vi "WLAN Tx Test Get Default USL.vi"(8 "error in (no error)":errorcluster, 11 "Template Tx Test in":refnum<class "niDTS WLAN Tx Test.lvclass">) -> (0 "error out":errorcluster, 2 "Default USL":T1 {"OBW"."Stop Frequency (Hz)" format="%#_4p"; "OBW"."Start Frequency (Hz)" format="%#_4p"; "OBW"."OBW (Hz)" format="%#_4p"}, 3 "Template Tx Test out":refnum<class "niDTS WLAN Tx Test.lvclass">)   [LabVIEW 2015, in "niDTS WLAN.lvlib" / "niDTS WLAN Tx Test.lvclass"]
uses:
  niDTS WLAN Tx Test.lvclass
  Includes/niDTS WLAN Tx Test INC Results.ctl
  Includes/niDTS WLAN Tx Test INC MOD EVM Results.ctl
  Includes/Results/niDTS Tx RES INC EVM.ctl
  Includes/niDTS WLAN Tx Test INC TXP Results.ctl
  Includes/niDTS WLAN Tx Test INC TXP Result SINGLE.ctl
  Includes/niDTS WLAN Tx Test INC OBW Results.ctl
  Instrument/INSTR TX/Results/niDTS WLAN INSTR TX INC SEM Results.ctl
  Instrument/INSTR TX/Results/niDTS WLAN INSTR TX INC SEM FSEGemts Results.ctl
  Includes/Results/niDTS Tx RES INC SEM FSEGemts.ctl
  Instrument/INSTR TX/Results/niDTS WLAN INSTR TX INC SEM MARGin Results.ctl
  Includes/Results/niDTS Tx RES INC SEM Margin.ctl
  Instrument/INSTR TX/Results/niDTS WLAN INSTR TX INC OFDM Impairments Results.ctl
  niDTS WLAN Tx Test.lvclass/niDTS WLAN Tx Test.ctl
  Includes/niDTS WLAN Tx Test INC Default Limits.vi
  niDTS WLAN.lvlib
  Instrument/INSTR TX/niDTS WLAN INSTR TX.lvclass
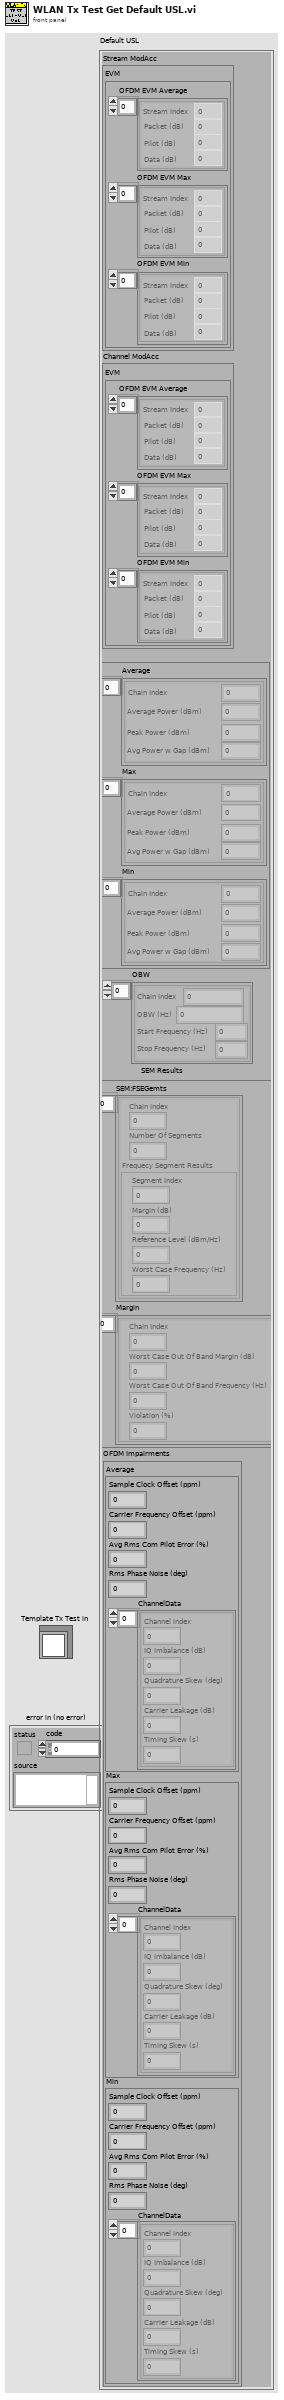
[diagram p1: front panel]
types:
  T1 = typedef "niDTS WLAN.lvlib/niDTS WLAN Tx Test INC Results.ctl" = cluster{"Stream ModAcc":T2, "Channel ModAcc":T2, "TXP":T4, "OBW":T6[], "SEM Results":T7, "OFDM Impairments":T12}
  T2 = typedef "niDTS WLAN.lvlib/niDTS WLAN Tx Test INC MOD EVM Results.ctl" = cluster{"EVM":cluster{"OFDM EVM Average":T3[], "OFDM EVM Max":T3[], "OFDM EVM Min":T3[]}}
  T3 = typedef "niDTS WLAN.lvlib/niDTS Tx RES INC EVM.ctl" = cluster{"Stream Index":i32, "Packet (dB)":dbl, "Pilot (dB)":dbl, "Data (dB)":dbl}
  T4 = typedef "niDTS WLAN.lvlib/niDTS WLAN Tx Test INC TXP Results.ctl" = cluster{"Average":T5[], "Max":T5[], "Min":T5[]}
  T5 = typedef "niDTS WLAN.lvlib/niDTS WLAN Tx Test INC TXP Result SINGLE.ctl" = cluster{"Chain Index":dbl, "Average Power (dBm)":dbl, "Peak Power (dBm)":dbl, "Avg Power w Gap (dBm)":dbl}
  T6 = typedef "niDTS WLAN.lvlib/niDTS WLAN Tx Test INC OBW Results.ctl" = cluster{"Chain Index":dbl, "OBW (Hz)":dbl, "Start Frequency (Hz)":dbl, "Stop Frequency (Hz)":dbl}
  T7 = typedef "niDTS WLAN.lvlib/niDTS WLAN INSTR TX.lvclass/niDTS WLAN INSTR TX INC SEM Results.ctl" = cluster{"SEM:FSEGemts":T8, "Margin":T10}
  T8 = typedef "niDTS WLAN.lvlib/niDTS WLAN INSTR TX.lvclass/niDTS WLAN INSTR TX INC SEM FSEGemts Results.ctl" = T9[]
  T9 = typedef "niDTS WLAN.lvlib/niDTS Tx RES INC SEM FSEGemts.ctl" = cluster{"Chain Index":i32, "Number Of Segments":i32, "Frequecy Segment Results":cluster{"Segment Index":i32, "Margin (dB)":dbl, "Reference Level (dBm/Hz)":dbl, "Worst Case Frequency (Hz)":dbl}}
  T10 = typedef "niDTS WLAN.lvlib/niDTS WLAN INSTR TX.lvclass/niDTS WLAN INSTR TX INC SEM MARGin Results.ctl" = T11[]
  T11 = typedef "niDTS WLAN.lvlib/niDTS Tx RES INC SEM Margin.ctl" = cluster{"Chain Index":i32, "Worst Case Out Of Band Margin (dB)":dbl, "Worst Case Out Of Band Frequency (Hz)":dbl, "Violation (%)":dbl}
  T12 = typedef "niDTS WLAN.lvlib/niDTS WLAN INSTR TX.lvclass/niDTS WLAN INSTR TX INC OFDM Impairments Results.ctl" = cluster{"Average":cluster{"Sample Clock Offset (ppm)":dbl, "Carrier Frequency Offset (ppm)":dbl, "Avg Rms Com Pilot Error (%)":dbl, "Rms Phase Noise (deg)":dbl, "ChannelData":cluster{"Channel Index":i32, "IQ Imbalance (dB)":dbl, "Quadrature Skew (deg)":dbl, "Carrier Leakage (dB)":dbl, "Timing Skew (s)":dbl}[]}, "Max":cluster{"Sample Clock Offset (ppm)":dbl, "Carrier Frequency Offset (ppm)":dbl, "Avg Rms Com Pilot Error (%)":dbl, "Rms Phase Noise (deg)":dbl, "ChannelData":cluster{"Channel Index":i32, "IQ Imbalance (dB)":dbl, "Quadrature Skew (deg)":dbl, "Carrier Leakage (dB)":dbl, "Timing Skew (s)":dbl}[]}, "Min":cluster{"Sample Clock Offset (ppm)":dbl, "Carrier Frequency Offset (ppm)":dbl, "Avg Rms Com Pilot Error (%)":dbl, "Rms Phase Noise (deg)":dbl, "ChannelData":cluster{"Channel Index":i32, "IQ Imbalance (dB)":dbl, "Quadrature Skew (deg)":dbl, "Carrier Leakage (dB)":dbl, "Timing Skew (s)":dbl}[]}}
  T13 = cluster{"OFDM EVM Average":T3[], "OFDM EVM Max":T3[], "OFDM EVM Min":T3[]}
  T14 = typedef "niDTS WLAN.lvlib/niDTS WLAN INC Standard.ctl" = enum16{"802.11 b DSSS", "802.11 a/g OFDM", "802.11 n HT", "802.11 ac VHT"}
  T15 = typedef "niDTS WLAN.lvlib/niDTS WLAN INC CH BW.ctl" = enum16{"20 MHz", "40 MHz", "80 MHz", "160 MHz"}
  T16 = cluster{"SampleClockOffset":dbl, "CarrierFrequencyOffset":dbl, "AvgRmsComPilotErr":dbl, "RmsPhaseNoise":dbl, "ChannelData":cluster{"CarrierFrequencyOffset":i32, "AvgRmsComPilotErr":dbl, "RmsPhaseNoise":dbl, "ChannelData":dbl, "ChannelIndex":dbl}[]}
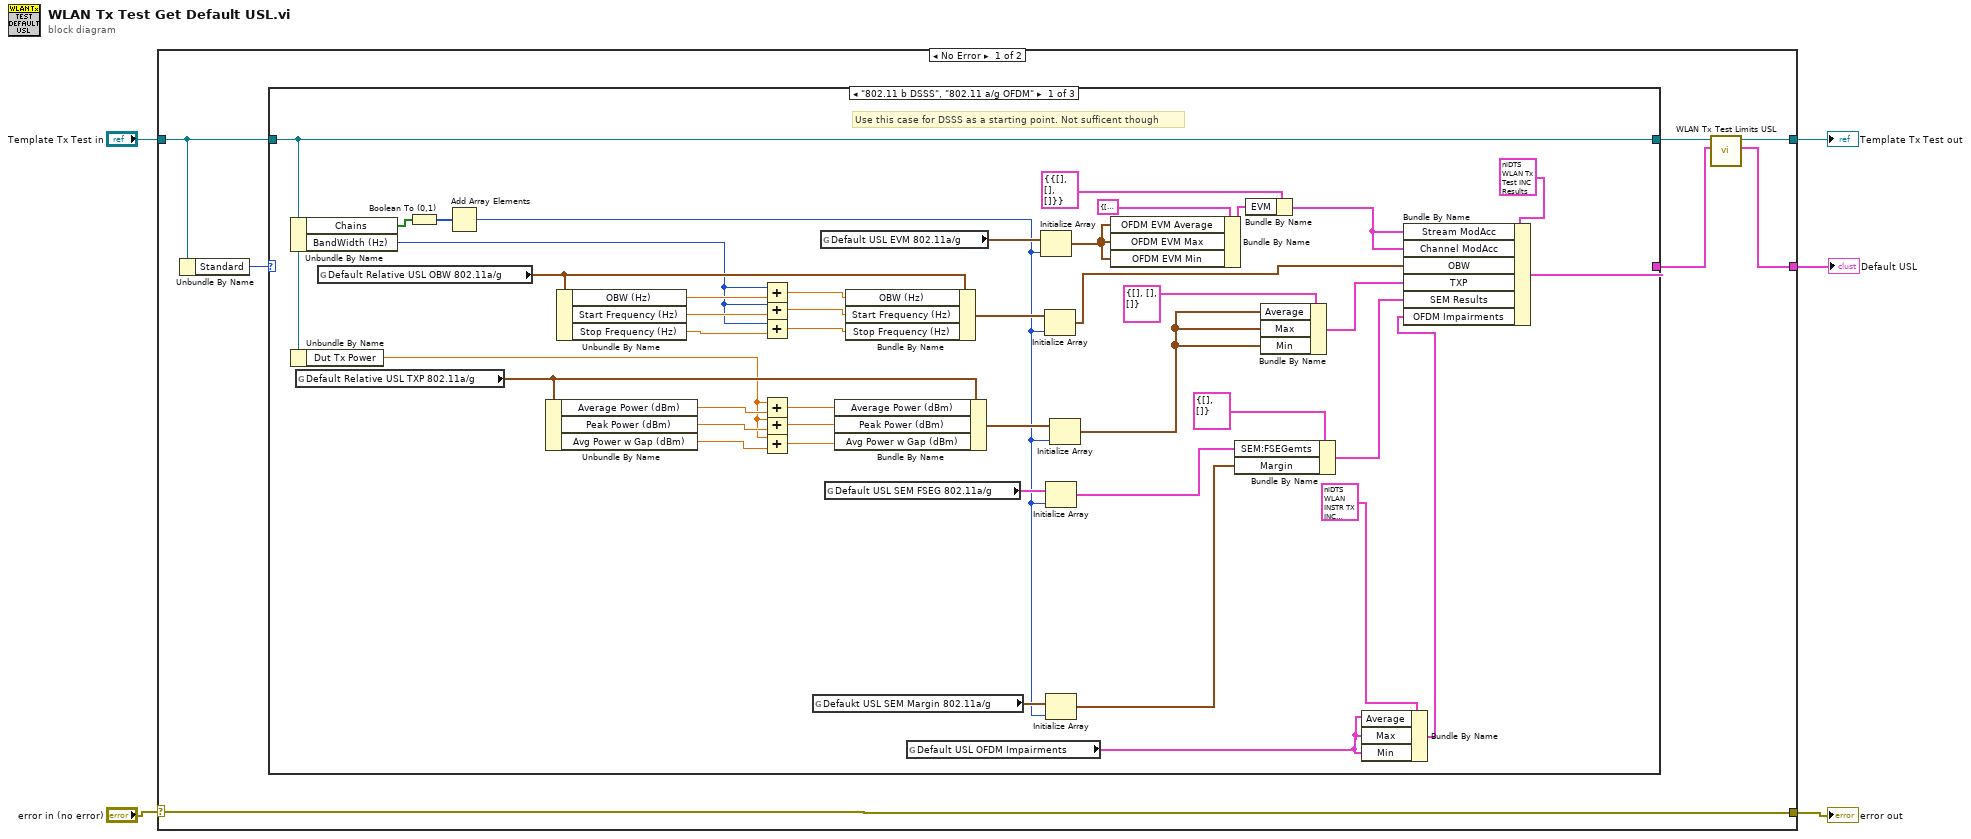
[diagram p0: block diagram]
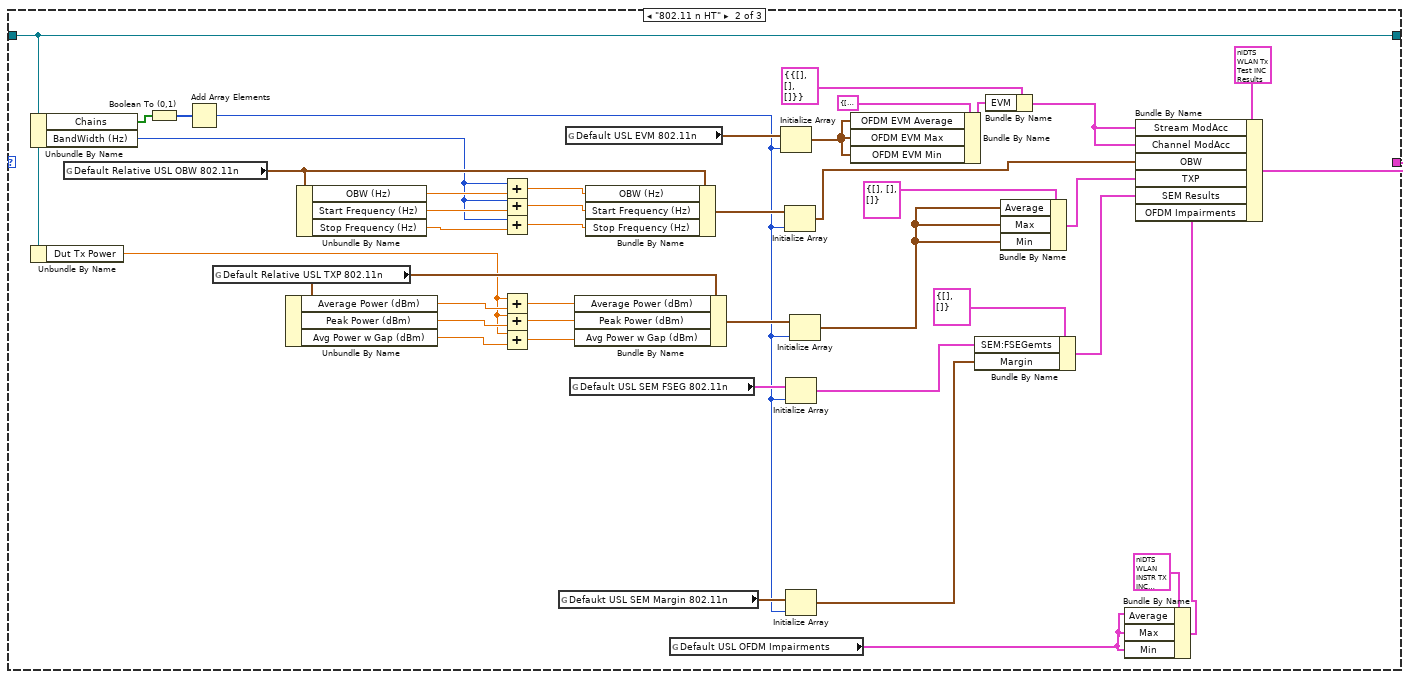
[diagram p2: hidden frame]
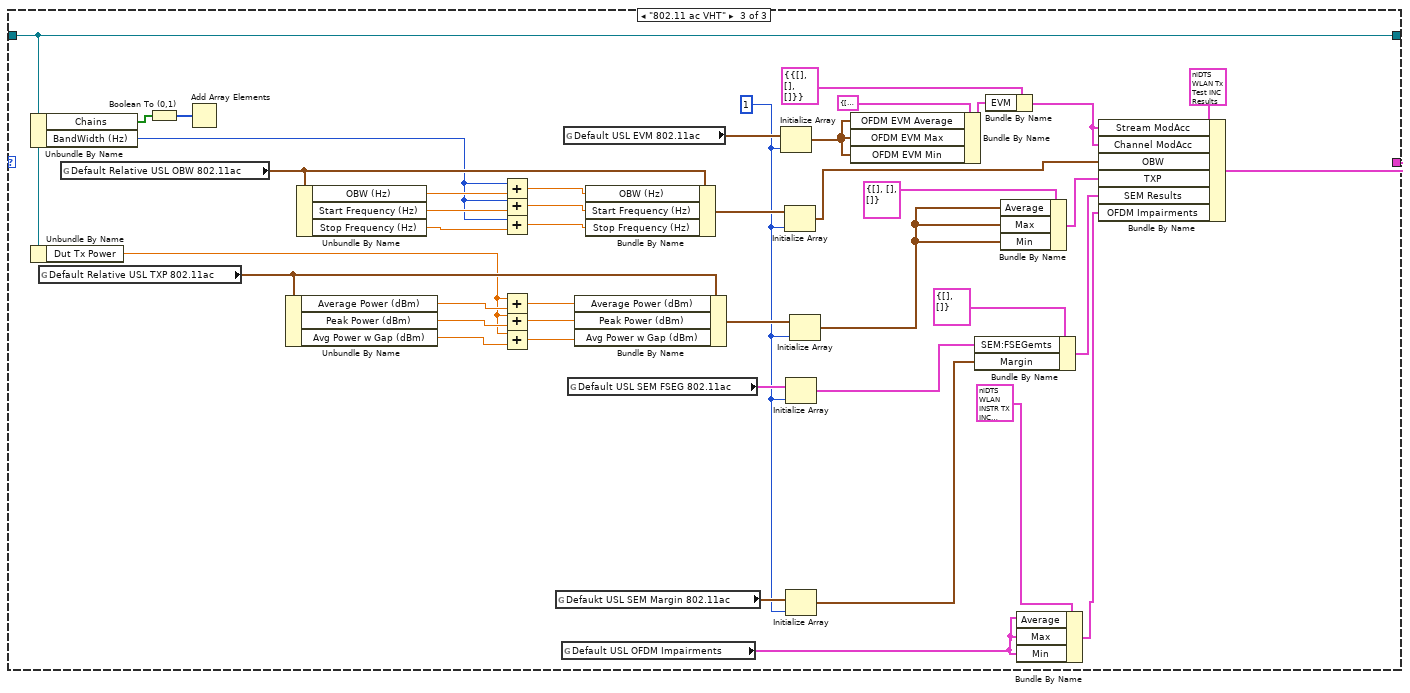
[diagram p3: hidden frame]
diagram:
  n1 = case shown="No Error" "error in (no error)" {
    selector: "error in (no error)" -> [w12 w143]
    tunnel: [w12 w143] -> w2
    tunnel: [w8 w142] -> w4
    tunnel: "Template Tx Test in" -> [w10 w142]
    tunnel: [w6 _] -> w1
    frame No Error {
      n2 = Unbundle By Name(w10) -> ("Standard"=w11:T14)
      n3 = case shown="\"802.11 b DSSS\", \"802.11 a/g OFDM\"" w11 {
        tunnel: [w54 w56 w140] -> w7
        tunnel: w10 -> [w45 w89 w131]
        tunnel: [w45 w89 w131] -> w9
        frame "802.11 b DSSS", "802.11 a/g OFDM" {
          # "Use this case for DSSS as a starting point. Not sufficent though"
          n4 = Unbundle By Name(w45) -> ("Chains"=w35:bool[], "BandWidth (Hz)"=w46:T15)
          n5 = Unbundle By Name(w45) -> ("Dut Tx Power"=w37:dbl)
          n6 = global read "niDTS WLAN Tx Test INC Default Limits.vi" "Default Relative USL TXP 802.11a/g"() -> (w44:T5)
          n7 = global read "niDTS WLAN Tx Test INC Default Limits.vi" "Default Relative USL OBW 802.11a/g"() -> (w53:T6)
          n8 = Boolean To (0,1)(Boolean=w35) -> (0, 1=w36:i16[])
          n9 = Add Array Elements(numeric array=w36) -> (sum=w18:i16)
          n10 = Unbundle By Name(w44) -> ("Average Power (dBm)"=w43:dbl, "Peak Power (dBm)"=w39:dbl, "Avg Power w Gap (dBm)"=w38:dbl)
          n11 = Unbundle By Name(w53) -> ("OBW (Hz)"=w47:dbl, "Start Frequency (Hz)"=w49:dbl, "Stop Frequency (Hz)"=w48:dbl)
          n12 = Add(x=w46, y=w47) -> (x+y=w52:dbl)
          n13 = Add(x=w46, y=w49) -> (x+y=w51:dbl)
          n14 = Add(x=w46, y=w48) -> (x+y=w50:dbl)
          n15 = Add(x=w37, y=w43) -> (x+y=w42:dbl)
          n16 = Add(x=w37, y=w39) -> (x+y=w41:dbl)
          n17 = Add(x=w37, y=w38) -> (x+y=w40:dbl)
          n18 = global read "niDTS WLAN Tx Test INC Default Limits.vi" "Defaukt USL SEM Margin 802.11a/g"() -> (w19:T11)
          n19 = global read "niDTS WLAN Tx Test INC Default Limits.vi" "Default USL EVM 802.11a/g"() -> (w34:T3)
          n20 = global read "niDTS WLAN Tx Test INC Default Limits.vi" "Default USL SEM FSEG 802.11a/g"() -> (w21:T9)
          n21 = Bundle By Name(cluster=w44, "Average Power (dBm)"=w42, "Peak Power (dBm)"=w41, "Avg Power w Gap (dBm)"=w40) -> (w25:T5)
          n22 = Bundle By Name(cluster=w53, "OBW (Hz)"=w52, "Start Frequency (Hz)"=w51, "Stop Frequency (Hz)"=w50) -> (w28:T6)
          n23 = global read "niDTS WLAN Tx Test INC Default Limits.vi" "Default USL OFDM Impairments"() -> (w14:T16)
          n24 = Initialize Array(w34, w18) -> (w31:T3[])
          n25 = Initialize Array(w28, w18) -> (w23:T6[])
          n26 = Initialize Array(w21, w18) -> (w20:T9[])
          n27 = Initialize Array(w19, w18) -> (w17:T11[])
          n28 = Initialize Array(w25, w18) -> (w24:T5[])
          n29 = Bundle By Name(cluster=T13 {"OFDM EVM Average"=[], "OFDM EVM Max"=[], "OFDM EVM Min"=[]} ("EVM"), "OFDM EVM Average"=w31, "OFDM EVM Max"=w31, "OFDM EVM Min"=w31) -> (w30:T13)
          n30 = Bundle By Name(cluster=T7 {"SEM:FSEGemts"=[], "Margin"=[]} ("SEM Results"), "SEM:FSEGemts"=w20, "Margin"=w17) -> (w16:T7)
          n31 = Bundle By Name(cluster=T2 {"EVM"={"OFDM EVM Average"=[], "OFDM EVM Max"=[], "OFDM EVM Min"=[]}} ("Stream ModAcc"), "EVM"=w30) -> (w29:T2)
          n32 = Bundle By Name(cluster=T4 {"Average"=[], "Max"=[], "Min"=[]} ("TXP Results"), "Average"=w24, "Max"=w24, "Min"=w24) -> (w26:T4)
          n33 = Bundle By Name(cluster=T12 {"Average"={"Sample Clock Offset (ppm)"=0.0, "Carrier Frequency Offset (ppm)"=0.0, "Avg Rms Com Pilot Error (%)"=0.0, "Rms Phase Noise (deg)"=0.0, "ChannelData"=[]}, "Max"={"Sample Clock Offset (ppm)"=0.0, "Carrier Frequency Offset (ppm)"=0.0, "Avg Rms Com Pilot Error (%)"=0.0, "Rms Phase Noise (deg)"=0.0, "ChannelData"=[]}, "Min"={"Sample Clock Offset (ppm)"=0.0, "Carrier Frequency Offset (ppm)"=0.0, "Avg Rms Com Pilot Error (%)"=0.0, "Rms Phase Noise (deg)"=0.0, "ChannelData"=[]}} ("OFDM Impairments"), "Average"=w14, "Max"=w14, "Min"=w14) -> (w13:T12)
          n34 = Bundle By Name(cluster=T1 {"Stream ModAcc"={"EVM"={"OFDM EVM Average"=[], "OFDM EVM Max"=[], "OFDM EVM Min"=[]}}, "Channel ModAcc"={"EVM"={"OFDM EVM Average"=[], "OFDM EVM Max"=[], "OFDM EVM Min"=[]}}, "TXP"={"Average"=[], "Max"=[], "Min"=[]}, "OBW"=[], "SEM Results"={"SEM:FSEGemts"=[], "Margin"=[]}, "OFDM Impairments"={"Average"={"Sample Clock Offset (ppm)"=0.0, "Carrier Frequency Offset (ppm)"=0.0, "Avg Rms Com Pilot Error (%)"=0.0, "Rms Phase Noise (deg)"=0.0, "ChannelData"=[]}, "Max"={"Sample Clock Offset (ppm)"=0.0, "Carrier Frequency Offset (ppm)"=0.0, "Avg Rms Com Pilot Error (%)"=0.0, "Rms Phase Noise (deg)"=0.0, "ChannelData"=[]}, "Min"={"Sample Clock Offset (ppm)"=0.0, "Carrier Frequency Offset (ppm)"=0.0, "Avg Rms Com Pilot Error (%)"=0.0, "Rms Phase Noise (deg)"=0.0, "ChannelData"=[]}}} ("Default USL"), "Stream ModAcc"=w29, "Channel ModAcc"=w29, "OBW"=w23, "TXP"=w26, "SEM Results"=w16, "OFDM Impairments"=w13) -> (w54:T1)
        }
        frame "802.11 n HT" {
          n35 = Unbundle By Name(w89) -> ("Chains"=w79:bool[], "BandWidth (Hz)"=w90:T15)
          n36 = Unbundle By Name(w89) -> ("Dut Tx Power"=w81:dbl)
          n37 = global read "niDTS WLAN Tx Test INC Default Limits.vi" "Default Relative USL OBW 802.11n"() -> (w97:T6)
          n38 = Boolean To (0,1)(Boolean=w79) -> (0, 1=w80:i16[])
          n39 = Add Array Elements(numeric array=w80) -> (sum=w62:i16)
          n40 = global read "niDTS WLAN Tx Test INC Default Limits.vi" "Default Relative USL TXP 802.11n"() -> (w88:T5)
          n41 = Unbundle By Name(w88) -> ("Average Power (dBm)"=w87:dbl, "Peak Power (dBm)"=w83:dbl, "Avg Power w Gap (dBm)"=w82:dbl)
          n42 = Unbundle By Name(w97) -> ("OBW (Hz)"=w91:dbl, "Start Frequency (Hz)"=w93:dbl, "Stop Frequency (Hz)"=w92:dbl)
          n43 = Add(x=w90, y=w91) -> (x+y=w96:dbl)
          n44 = Add(x=w90, y=w93) -> (x+y=w95:dbl)
          n45 = Add(x=w90, y=w92) -> (x+y=w94:dbl)
          n46 = Add(x=w81, y=w87) -> (x+y=w86:dbl)
          n47 = Add(x=w81, y=w83) -> (x+y=w85:dbl)
          n48 = Add(x=w81, y=w82) -> (x+y=w84:dbl)
          n49 = global read "niDTS WLAN Tx Test INC Default Limits.vi" "Defaukt USL SEM Margin 802.11n"() -> (w63:T11)
          n50 = global read "niDTS WLAN Tx Test INC Default Limits.vi" "Default USL EVM 802.11n"() -> (w78:T3)
          n51 = global read "niDTS WLAN Tx Test INC Default Limits.vi" "Default USL SEM FSEG 802.11n"() -> (w65:T9)
          n52 = Bundle By Name(cluster=w88, "Average Power (dBm)"=w86, "Peak Power (dBm)"=w85, "Avg Power w Gap (dBm)"=w84) -> (w69:T5)
          n53 = Bundle By Name(cluster=w97, "OBW (Hz)"=w96, "Start Frequency (Hz)"=w95, "Stop Frequency (Hz)"=w94) -> (w72:T6)
          n54 = global read "niDTS WLAN Tx Test INC Default Limits.vi" "Default USL OFDM Impairments"() -> (w58:T16)
          n55 = Initialize Array(w78, w62) -> (w75:T3[])
          n56 = Initialize Array(w72, w62) -> (w67:T6[])
          n57 = Initialize Array(w65, w62) -> (w64:T9[])
          n58 = Initialize Array(w63, w62) -> (w61:T11[])
          n59 = Initialize Array(w69, w62) -> (w68:T5[])
          n60 = Bundle By Name(cluster=T13 {"OFDM EVM Average"=[], "OFDM EVM Max"=[], "OFDM EVM Min"=[]} ("EVM"), "OFDM EVM Average"=w75, "OFDM EVM Max"=w75, "OFDM EVM Min"=w75) -> (w74:T13)
          n61 = Bundle By Name(cluster=T7 {"SEM:FSEGemts"=[], "Margin"=[]} ("SEM Results"), "SEM:FSEGemts"=w64, "Margin"=w61) -> (w60:T7)
          n62 = Bundle By Name(cluster=T2 {"EVM"={"OFDM EVM Average"=[], "OFDM EVM Max"=[], "OFDM EVM Min"=[]}} ("Stream ModAcc"), "EVM"=w74) -> (w73:T2)
          n63 = Bundle By Name(cluster=T4 {"Average"=[], "Max"=[], "Min"=[]} ("TXP Results"), "Average"=w68, "Max"=w68, "Min"=w68) -> (w70:T4)
          n64 = Bundle By Name(cluster=T12 {"Average"={"Sample Clock Offset (ppm)"=0.0, "Carrier Frequency Offset (ppm)"=0.0, "Avg Rms Com Pilot Error (%)"=0.0, "Rms Phase Noise (deg)"=0.0, "ChannelData"=[]}, "Max"={"Sample Clock Offset (ppm)"=0.0, "Carrier Frequency Offset (ppm)"=0.0, "Avg Rms Com Pilot Error (%)"=0.0, "Rms Phase Noise (deg)"=0.0, "ChannelData"=[]}, "Min"={"Sample Clock Offset (ppm)"=0.0, "Carrier Frequency Offset (ppm)"=0.0, "Avg Rms Com Pilot Error (%)"=0.0, "Rms Phase Noise (deg)"=0.0, "ChannelData"=[]}} ("OFDM Impairments"), "Average"=w58, "Max"=w58, "Min"=w58) -> (w57:T12)
          n65 = Bundle By Name(cluster=T1 {"Stream ModAcc"={"EVM"={"OFDM EVM Average"=[], "OFDM EVM Max"=[], "OFDM EVM Min"=[]}}, "Channel ModAcc"={"EVM"={"OFDM EVM Average"=[], "OFDM EVM Max"=[], "OFDM EVM Min"=[]}}, "TXP"={"Average"=[], "Max"=[], "Min"=[]}, "OBW"=[], "SEM Results"={"SEM:FSEGemts"=[], "Margin"=[]}, "OFDM Impairments"={"Average"={"Sample Clock Offset (ppm)"=0.0, "Carrier Frequency Offset (ppm)"=0.0, "Avg Rms Com Pilot Error (%)"=0.0, "Rms Phase Noise (deg)"=0.0, "ChannelData"=[]}, "Max"={"Sample Clock Offset (ppm)"=0.0, "Carrier Frequency Offset (ppm)"=0.0, "Avg Rms Com Pilot Error (%)"=0.0, "Rms Phase Noise (deg)"=0.0, "ChannelData"=[]}, "Min"={"Sample Clock Offset (ppm)"=0.0, "Carrier Frequency Offset (ppm)"=0.0, "Avg Rms Com Pilot Error (%)"=0.0, "Rms Phase Noise (deg)"=0.0, "ChannelData"=[]}}} ("Default USL"), "Stream ModAcc"=w73, "Channel ModAcc"=w73, "OBW"=w67, "TXP"=w70, "SEM Results"=w60, "OFDM Impairments"=w57) -> (w56:T1)
        }
        frame "802.11 ac VHT" {
          w102 = 1
          n66 = Unbundle By Name(w131) -> ("Chains"=w121:bool[], "BandWidth (Hz)"=w132:T15)
          n67 = Unbundle By Name(w131) -> ("Dut Tx Power"=w123:dbl)
          n68 = global read "niDTS WLAN Tx Test INC Default Limits.vi" "Default Relative USL TXP 802.11ac"() -> (w130:T5)
          n69 = global read "niDTS WLAN Tx Test INC Default Limits.vi" "Default Relative USL OBW 802.11ac"() -> (w139:T6)
          n70 = Boolean To (0,1)(Boolean=w121) -> (0, 1=w122:i16[])
          n71 = Add Array Elements(numeric array=w122) -> ()  [unwired: 1 out]
          n72 = Unbundle By Name(w130) -> ("Average Power (dBm)"=w129:dbl, "Peak Power (dBm)"=w125:dbl, "Avg Power w Gap (dBm)"=w124:dbl)
          n73 = Unbundle By Name(w139) -> ("OBW (Hz)"=w133:dbl, "Start Frequency (Hz)"=w135:dbl, "Stop Frequency (Hz)"=w134:dbl)
          n74 = Add(x=w132, y=w133) -> (x+y=w138:dbl)
          n75 = Add(x=w132, y=w135) -> (x+y=w137:dbl)
          n76 = Add(x=w132, y=w134) -> (x+y=w136:dbl)
          n77 = Add(x=w123, y=w129) -> (x+y=w128:dbl)
          n78 = Add(x=w123, y=w125) -> (x+y=w127:dbl)
          n79 = Add(x=w123, y=w124) -> (x+y=w126:dbl)
          n80 = global read "niDTS WLAN Tx Test INC Default Limits.vi" "Defaukt USL SEM Margin 802.11ac"() -> (w105:T11)
          n81 = global read "niDTS WLAN Tx Test INC Default Limits.vi" "Default USL OFDM Impairments"() -> (w100:T16)
          n82 = global read "niDTS WLAN Tx Test INC Default Limits.vi" "Default USL EVM 802.11ac"() -> (w120:T3)
          n83 = global read "niDTS WLAN Tx Test INC Default Limits.vi" "Default USL SEM FSEG 802.11ac"() -> (w107:T9)
          n84 = Bundle By Name(cluster=w130, "Average Power (dBm)"=w128, "Peak Power (dBm)"=w127, "Avg Power w Gap (dBm)"=w126) -> (w111:T5)
          n85 = Bundle By Name(cluster=w139, "OBW (Hz)"=w138, "Start Frequency (Hz)"=w137, "Stop Frequency (Hz)"=w136) -> (w114:T6)
          n86 = Initialize Array(w120, w102) -> (w117:T3[])
          n87 = Initialize Array(w114, w102) -> (w109:T6[])
          n88 = Initialize Array(w107, w102) -> (w106:T9[])
          n89 = Initialize Array(w105, w102) -> (w104:T11[])
          n90 = Initialize Array(w111, w102) -> (w110:T5[])
          n91 = Bundle By Name(cluster=T13 {"OFDM EVM Average"=[], "OFDM EVM Max"=[], "OFDM EVM Min"=[]} ("EVM"), "OFDM EVM Average"=w117, "OFDM EVM Max"=w117, "OFDM EVM Min"=w117) -> (w116:T13)
          n92 = Bundle By Name(cluster=T7 {"SEM:FSEGemts"=[], "Margin"=[]} ("SEM Results"), "SEM:FSEGemts"=w106, "Margin"=w104) -> (w103:T7)
          n93 = Bundle By Name(cluster=T2 {"EVM"={"OFDM EVM Average"=[], "OFDM EVM Max"=[], "OFDM EVM Min"=[]}} ("Stream ModAcc"), "EVM"=w116) -> (w115:T2)
          n94 = Bundle By Name(cluster=T4 {"Average"=[], "Max"=[], "Min"=[]} ("TXP Results"), "Average"=w110, "Max"=w110, "Min"=w110) -> (w112:T4)
          n95 = Bundle By Name(cluster=T12 {"Average"={"Sample Clock Offset (ppm)"=0.0, "Carrier Frequency Offset (ppm)"=0.0, "Avg Rms Com Pilot Error (%)"=0.0, "Rms Phase Noise (deg)"=0.0, "ChannelData"=[]}, "Max"={"Sample Clock Offset (ppm)"=0.0, "Carrier Frequency Offset (ppm)"=0.0, "Avg Rms Com Pilot Error (%)"=0.0, "Rms Phase Noise (deg)"=0.0, "ChannelData"=[]}, "Min"={"Sample Clock Offset (ppm)"=0.0, "Carrier Frequency Offset (ppm)"=0.0, "Avg Rms Com Pilot Error (%)"=0.0, "Rms Phase Noise (deg)"=0.0, "ChannelData"=[]}} ("OFDM Impairments"), "Average"=w100, "Max"=w100, "Min"=w100) -> (w99:T12)
          n96 = Bundle By Name(cluster=T1 {"Stream ModAcc"={"EVM"={"OFDM EVM Average"=[], "OFDM EVM Max"=[], "OFDM EVM Min"=[]}}, "Channel ModAcc"={"EVM"={"OFDM EVM Average"=[], "OFDM EVM Max"=[], "OFDM EVM Min"=[]}}, "TXP"={"Average"=[], "Max"=[], "Min"=[]}, "OBW"=[], "SEM Results"={"SEM:FSEGemts"=[], "Margin"=[]}, "OFDM Impairments"={"Average"={"Sample Clock Offset (ppm)"=0.0, "Carrier Frequency Offset (ppm)"=0.0, "Avg Rms Com Pilot Error (%)"=0.0, "Rms Phase Noise (deg)"=0.0, "ChannelData"=[]}, "Max"={"Sample Clock Offset (ppm)"=0.0, "Carrier Frequency Offset (ppm)"=0.0, "Avg Rms Com Pilot Error (%)"=0.0, "Rms Phase Noise (deg)"=0.0, "ChannelData"=[]}, "Min"={"Sample Clock Offset (ppm)"=0.0, "Carrier Frequency Offset (ppm)"=0.0, "Avg Rms Com Pilot Error (%)"=0.0, "Rms Phase Noise (deg)"=0.0, "ChannelData"=[]}}} ("Default USL"), "Stream ModAcc"=w115, "Channel ModAcc"=w115, "OBW"=w109, "TXP"=w112, "SEM Results"=w103, "OFDM Impairments"=w99) -> (w140:T1)
        }
      }
      n97 = call-dynamic "WLAN Tx Test Limits USL.vi"("Limits"=w7, "WLAN Tx Test in"=w9) -> ("Limits Out"=w6:T1, "WLAN Tx Test out"=w8:refnum<class "niDTS WLAN Tx Test.lvclass">)  [unwired: 7 in, 1 out]
    }
    frame Error {
    }
  }
  "error out" <- w2
  "Template Tx Test out" <- w4
  "Default USL" <- w1
